vi "Protocol Read.vi"(8 "error in (no error)":errorcluster, 9 "timeout":i32=10000, 10 "bytes to read":i32, 11 "protocol layer in":refnum<class "Serial Master.lvclass">) -> (0 "error out":errorcluster, 1 "timed out?":bool, 2 "data":u8[](array[numeric]), 3 "protocol layer out":refnum<class "Serial Master.lvclass">)   [LabVIEW 2015, in "SubVIs.lvlib" / "Serial Master.lvclass"]
doc: "This provides an interface for reading from a network bus."
uses:
  <vilib>/Modbus/subvis/Protocol/Serial/Serial Master/Serial Master.lvclass
  <vilib>/Modbus/subvis/Protocol/Serial/Serial Master/Serial Master.lvclass/Serial Master.ctl
  <vilib>/Modbus/subvis/Protocol/Serial/Serial Shared Components/Serial Shared Components.lvlib
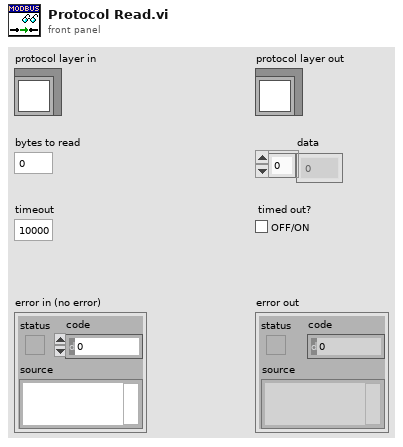
[diagram p1: front panel]
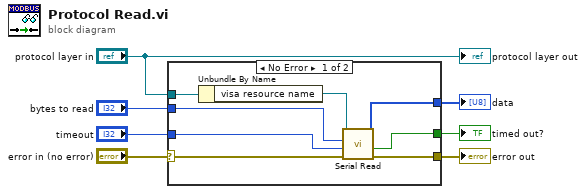
[diagram p0: block diagram]
diagram:
  n1 = case shown="No Error" "error in (no error)" {
    selector: "error in (no error)" -> [w8 w16]
    tunnel: "protocol layer in" -> [w14 _]
    tunnel: "bytes to read" -> [w13 _]
    tunnel: "timeout" -> [w12 _]
    tunnel: [w11 _] -> w4
    tunnel: [w10 _] -> w3
    tunnel: [w9 w16] -> w2
    frame No Error {
      n2 = Unbundle By Name(w14) -> ("visa resource name"=w15:refnum<visa-resource-name>)
      n3 = call <vilib>:"Serial Read.vi"("error in (no error)"=w8, "timeout (ms)"=w12, "bytes to read"=w13, "VISA resource"=w15) -> ("error out"=w9:errorcluster, "timed out?"=w11:bool, "data"=w10:u8[])  [unwired: 5 in]
    }
    frame Error {
    }
  }
  "error out" <- w2
  "data" <- w3
  "timed out?" <- w4
  "protocol layer out" <- "protocol layer in"
